vi "Fill Display.vi"(8 "error in (no error)":errorcluster, 10 "Color":u32(colorbox), 11 "RPI.SenseHat.Actor in":refnum<class "RPI.SenseHat.Actor.lvclass">) -> (0 "error out":errorcluster, 3 "RPI.SenseHat.Actor out":refnum<class "RPI.SenseHat.Actor.lvclass">)   [LabVIEW 2020, in "RPI.SenseHat.Actor.lvlib" / "RPI.SenseHat.Actor.lvclass"]
uses:
  RPI.SenseHat.Actor.lvclass
  RPI.SenseHat.Actor.lvclass/RPI.SenseHat.Actor.ctl
  RPI.SenseHat/SenseHat/SenseHat.lvclass/SenseHat.ctl
  RPI.SenseHat/SenseHat/Get RPI.SenseHat.Display.vi
  RPI.SenseHat.Display/Classes/SenseHat.Display/RPI.SenseHat.Display.lvclass
  RPI.SenseHat.Display/Classes/Color/Color.lvclass
  RPI.SenseHat/SenseHat/SenseHat.lvclass
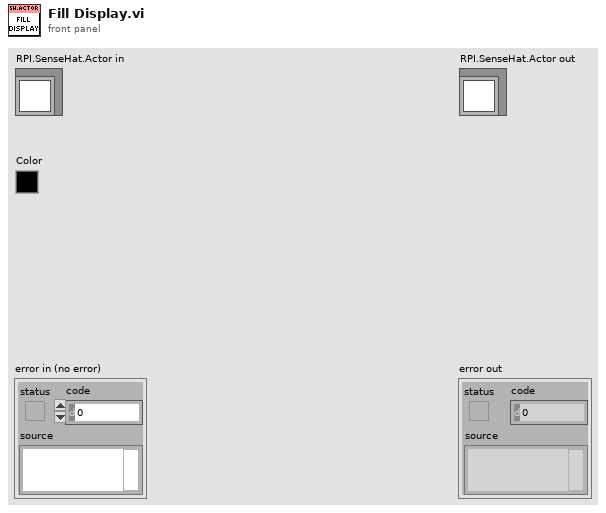
[diagram p1: front panel]
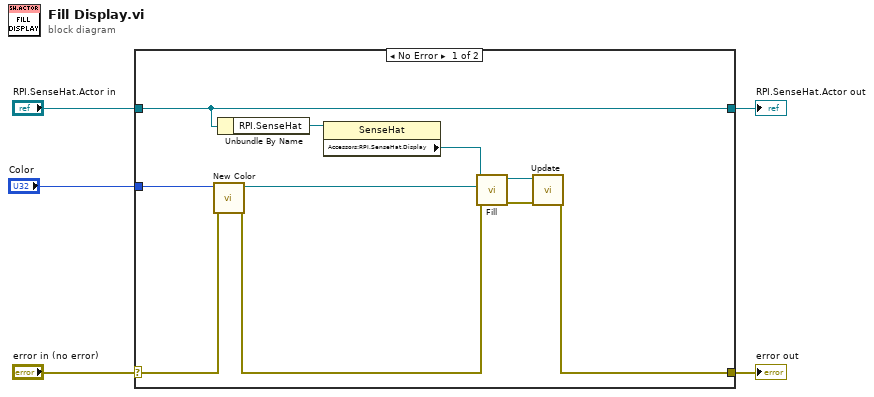
[diagram p0: block diagram]
diagram:
  n1 = case shown="No Error" "error in (no error)" {
    selector: "error in (no error)" -> [w8 w17]
    tunnel: [w6 w17] -> w4
    tunnel: [w9 w16] -> w2
    tunnel: "RPI.SenseHat.Actor in" -> [w9 w16]
    tunnel: "Color" -> [w10 _]
    frame No Error {
      n2 = call "New Color.vi"("error in (no error)"=w8, "Color Box"=w10) -> ("error out"=w7:errorcluster, "Color out"=w11:refnum<class "Color.lvclass">)  [unwired: 8 in]
      n3 = Unbundle By Name(w9) -> ("RPI.SenseHat"=w15:refnum<class "SenseHat.lvclass">)
      n4 = property class="SenseHat"(reference=w15) -> ("Accessors:RPI.SenseHat.Display"=w14:refnum<class "RPI.SenseHat.Display.lvclass">)  [unwired: 1 in, 2 out]
      n5 = call "Fill.vi"("error in (no error)"=w7, "Color"=w11, "senseHatDisplay in"=w14) -> ("error out"=w12:errorcluster, "senseHatDisplay out"=w13:refnum<class "RPI.SenseHat.Display.lvclass">)  [unwired: 7 in]
      n6 = call "Update.vi"("error in (no error)"=w12, "senseHatDisplay in"=w13) -> ("error out"=w6:errorcluster)  [unwired: 8 in, 1 out]
    }
    frame Error {
    }
  }
  "error out" <- w4
  "RPI.SenseHat.Actor out" <- w2
